vi "testgraphe.vi"() -> ()   [LabVIEW 2010]
panel:
  out "XY Graph":cluster{"Y":dbl[], "Y":dbl[]}[](graph) caption="Graphe XY"
  in  "Input Table":string[][](array[string])
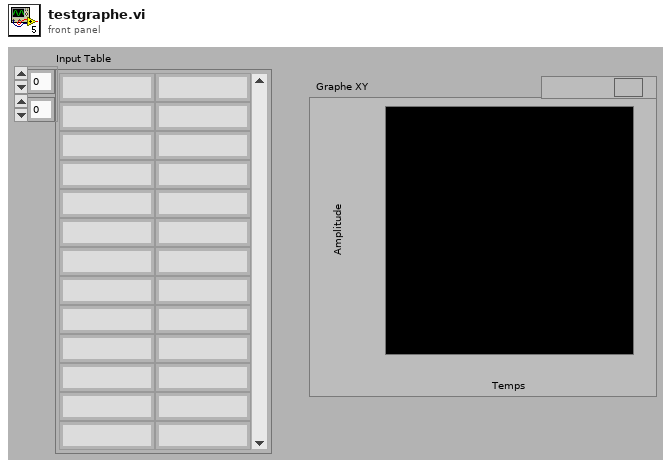
[diagram p1: front panel]
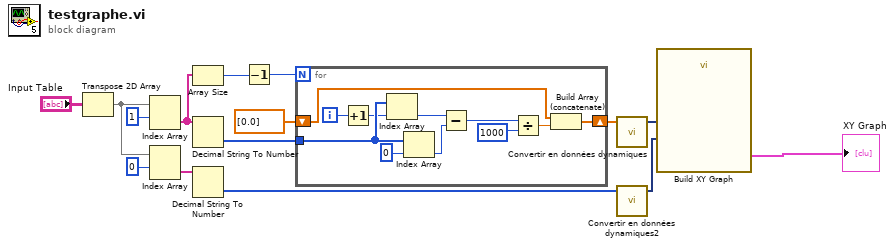
[diagram p0: block diagram]
diagram:
  n1 = Transpose 2D Array(2D array="Input Table") -> (transposed array=w13:string[][])
  n2 = Index Array(array=w13, index (row)=1 ("indice (ligne)")) -> (element=w6:string[])  [unwired: 1 in]
  n3 = Index Array(array=w13, index (row)=0 ("indice (ligne)")) -> (element=w15:string[])  [unwired: 1 in]
  n4 = Array Size(array=w6) -> (size(s)=w5:i32)
  n5 = Decimal String To Number(string=w6) -> (number=w8:i32[])  [unwired: 2 in, 1 out]
  n6 = Decimal String To Number(string=w15) -> (number=w3:i32[])  [unwired: 2 in, 1 out]
  n7 = Decrement(x=w5) -> (x-1=w4:i32)
  n8 = for {
    N: w4 -> [_]
    tunnel: w8 -> [w26]
    shift-right: [w16] -> w2
    shift-left: dbl[] [0.0] -> [w17]
    i -> [w25]
    n9 = Increment(x=w25) -> (x+1=w24:i32)
    n10 = Index Array(array=w26, index=w24) -> (element=w22:i32)
    n11 = Index Array(array=w26, index=0 ("indice")) -> (element=w21:i32)
    n12 = Subtract(x=w22, y=w21) -> (x-y=w20:i32)
    n13 = Divide(x=w20, y=1000) -> (x/y=w18:dbl)
    n14 = Build Array (concatenate)(w17, w18) -> (w16:dbl[])
  }
  n15 = call "Convertir en données dynamiques"("Array"=w2) -> ("Dynamic Data Type"=w1:dynamicdata)  [unwired: 3 in]
  n16 = call "Convertir en données dynamiques2"("Array"=w3) -> ("Dynamic Data Type"=w9:dynamicdata)  [unwired: 3 in]
  n17 = call "Build XY Graph"("Y Input"=w9, "X Input"=w1) -> ("XY Graph"=→"XY Graph":cluster{"Y":dbl[], "Y":dbl[]}[])  [unwired: 3 in, 6 out]
